vi "byte_array_to_bool_array.vi"(8 "error in (no error)":errorcluster, 10 "Byte array":u8[](array[numeric])) -> (0 "error out":errorcluster, 2 "Boolean array":bool[](array[boolean]))   [LabVIEW 2018, in "Inficon IC6.lvlib"]
doc: "Take an array of bytes and convert it to an array of booleans where each boolean corresponds to a bit in a byte.\n\nBytes are formatted so the most significant bit represents the first element of the boolean sub-array for the byte."
uses:
  <instrlib>/Inficon IC6/Inficon IC6.lvlib
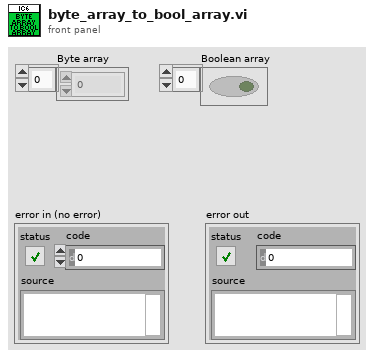
[diagram p1: front panel]
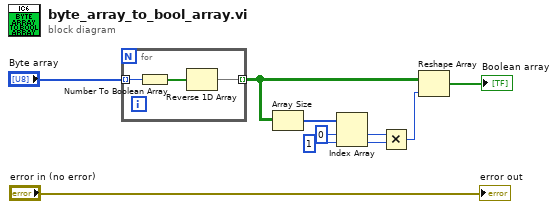
[diagram p0: block diagram]
diagram:
  n1 = for {
    tunnel: "Byte array" -> [w12] mode=indexing
    tunnel: [w11] -> w3 mode=indexing
    n2 = Number To Boolean Array(number=w12) -> (Boolean array=w13:bool[])
    n3 = Reverse 1D Array(array=w13) -> (reversed array=w11:bool[])
  }
  n4 = Array Size(array=w3) -> (size(s)=w4:i32[])
  n5 = Index Array(array=w4, index #1=0 ("index"), index #2=1 ("index")) -> (element #1=w7:i32, element #2=w8:i32)
  n6 = Multiply(x=w7, y=w8) -> (x*y=w9:i32)
  n7 = Reshape Array(w3, w9) -> (→"Boolean array":bool[])
  "error out" <- "error in (no error)"
